vi "Cycle Begin.vi"(8 "error in (no error)":errorcluster, 11 "Performance in":refnum<class "Performance.lvclass">) -> (0 "error out":errorcluster, 3 "Performance out":refnum<class "Performance.lvclass">)   [LabVIEW 2017, in "DSF Core.lvlib" / "Performance.lvclass"]
uses:
  Performance.lvclass
  Performance.lvclass/Performance.ctl
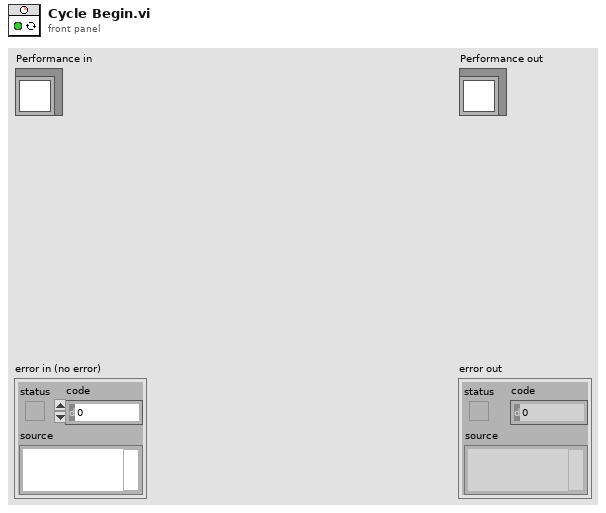
[diagram p1: front panel]
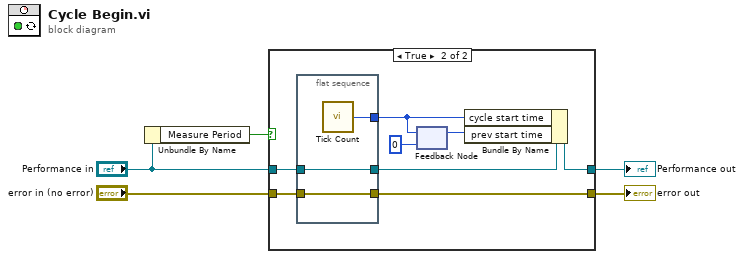
[diagram p0: block diagram]
diagram:
  n1 = Unbundle By Name("Performance in") -> ("Measure Period"=w1:bool)
  n2 = case shown="True" w1 {
    tunnel: [w6 w13] -> w5
    tunnel: "error in (no error)" -> [w6 w15]
    tunnel: [w7 w11] -> w3
    tunnel: "Performance in" -> [w7 w14]
    frame False {
    }
    frame True {
      n3 = flat-sequence {
        tunnel: w14 -> [w18]
        tunnel: w15 -> [w17]
        tunnel: [w18] -> w12
        tunnel: [w17] -> w13
        tunnel: [w16] -> w9
        frame #0 {
          n4 = call "Tick Count"() -> ("Tick Count(uSec)"=w16:u32)
        }
      }
      n5 = feedback-in #1(w9) -> ()
      n6 = feedback #1(u32 0 ("Tick Count(uSec)")) -> (w10:u32)
      n7 = Bundle By Name(cluster=w12, "cycle start time"=w9, "prev start time"=w10) -> (w11:refnum<class "Performance.lvclass">)
    }
  }
  "error out" <- w5
  "Performance out" <- w3
